vi "Saccade suppression - continuous flash LED.vi"() -> ()   [LabVIEW 2013]
uses:
  <vilib>/Platform/TimedLoop/XDataNode/timing_clust.ctl
  <vilib>/Platform/TimedLoop/XDataNode/nitl_modes.ctl
  <vilib>/Platform/TimedLoop/XDataNode/wakeup.ctl
  <vilib>/gmath/statdist.llb/Uniform (Discrete) Random.vi
  Eye tracking dependencies/Global 1.vi
  <vilib>/platform/TimedLoop/XDataNode/XDataNode.xnode
  <vilib>/Platform/TimedLoop/XDataNode/XDNodeRunTimeDep.lvlib
  <vilib>/gmath/NI_Gmath.lvlib
panel:
  out "Eye tracker":bool=TRUE
  out "Std name":string="70915_animal15-21_exp1"
  out "Blank":bool
  out "Total number of trials":i32=200
  out "Running!":bool
  in  "Location":string="D:\\Satoru\\Documents\\Attention_Beh_Data\\"
  out "File name exists!":bool
  out "Current trial #":u16
  out "LED":bool
  in  "Abort":bool caption="run-stop"
  in  "File name":string="animal15-29_exp1"
  in  "Save data":bool
  out "State Missed":bool
  out "VS missed":bool
  out "State busy":bool
  out "VS busy":bool
  in  "Tab Control":T1(tab)=enum."VS Parameters"
  in  "Notes":string
  in  "Start recording @":string
  in  "Inserted probe @":string
  in  "Brain region":string
  in  "Anesthesia @":string
  in  "Anesthesia":string
  in  "Probe configuration":string
  in  "Probe use number":string
  in  "Probe ID":string
  in  "Probe type":string
  in  "Electrode spacing":string
  in  "Electrode area":string
  in  "Penetration angle (to pia)":string
  in  "Penetration coordinates":string
  in  "Penetration distance":string
  in  "Penetration number":string
  in  "Genotype":string
  in  "Transfection":string
  in  "Mass":string
  in  "Sex":string
  in  "Age":string
  in  "Animal ID":string="14-4"
  in  "inter flash interval (ms)":dbl=300.0
  in  "Max jitter (ms)":dbl=250.0
  in  "VS type":string="continuous_flash"
  in  "Background luminance":sgl
  in  "Pulse amp 0":sgl
  in  "Pulse amp 1":sgl
  in  "Pulse delay (ms)":sgl
  in  "Pulse width (ms)":sgl
  in  "Pulse period":sgl
  in  "Pulse #":sgl
  in  "LED mode":u16(ring) items=["No LED", "Random"]
  in  "Chance (%)":dbl
  in  "# of trials":i32=200
  in  "run-stop":bool
  in  "movement":sgl=3.0
  in  "Flash luminance":sgl=100.0
  in  "flash duration (ms)":dbl=48.0
  in  "VS subtype":string="fullfield"
  in  "Include blanks":bool=TRUE
  in  "# of blank trials":i32=200
  in  "Give reward":bool
  in  "Manually give shock":bool
  in  "Water duration (ms)":u32=30
  in  "Shock duration (ms)":u32=10
  in  "Water refractory period (ms)":u32=500
  in  "Shock refractory period (ms)":u32=1000
  in  "Trial timeout (ms)":u32=3000
  in  "Track eye":bool=TRUE
  in  "Allow shock":bool
  in  "Allow timeout":bool
  in  "Manually give water":bool
  in  "Reward period (ms)":u32
  in  "Reward start delay (ms)":u32
  in  "Lick threshold (V)":fxp<+,32,16>=1.600006103515625
  in  "VS threshold (V)":fxp<+,32,16>=0.5
  out "Originating IP":string="192.168.137.2"
  out "Incoming data":string="TrlDone 1.000 "
  in  "Update cycle (ms)":dbl=50.0
  in  "Local IP_This computer":string="192.168.137.10"
  in  "Remote IP_Broadcast":string="192.168.137.255"
  in  "Remote IP_State machine":string="192.168.137.2"
  in  "Remote IP_Visual stimulation":string="192.168.137.3"
  in  "Local port":u16=9090
  in  "Remote port":u16=9091
  out "Error 2":string
  # "Saccade suppression project"
  # "Current trial"
  # "of"
  # "System Status"
  # "VS"
  # "State machine"
  # "Busy"
  # "Missed trial"
  # "Max 20 characters"
  # "(w/o LED)"
  # "Movement threshold (degrees)"
  # "MAX 199.9988"
  # "(% of blank trials that have LED)"
  # "Errors for debugging"
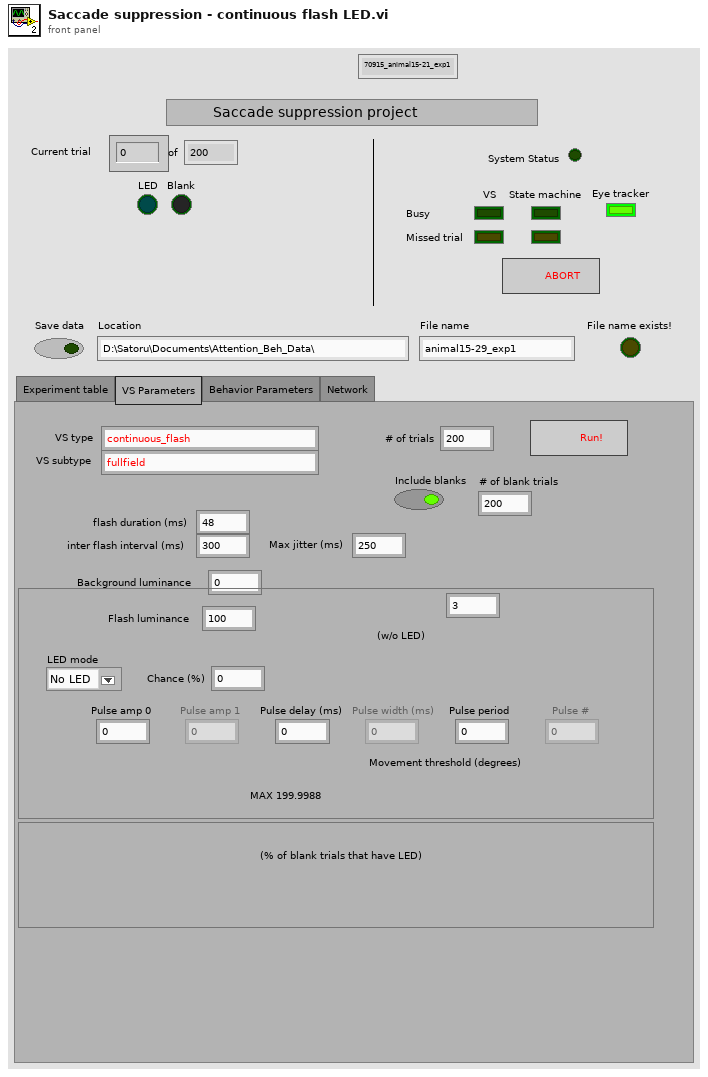
[diagram p1: front panel]
types:
  T1 = enum32{"Experiment table", "VS Parameters", "Behavior Parameters", "Network"}
  T2 = typedef "XDNodeRunTimeDep.lvlib/timing_clust.ctl" = cluster{"Expected End [f-1]":u64, "Actual End [f-1]":u64, "Finished Late? [f-1]":bool, "Expected End [i-1]":u64, "Actual End [i-1]":u64, "Finished Late? [i-1]":bool, "Expected Start [i]":u64, "Actual Start [i]":u64, "Expected Start [f]":u64, "Actual Start [f]":u64, "Source Name":string, "Structure Name":string, "Period":i64, "Deadline":i64, "Offset":i64, "Start":i64, "Priority":i32, "Timeout":i32, "Mode":T3, "Wakeup Reason":T4, "Error":errorcluster, "Source Type":string, "Secondary Source Type":string, "Global End Time":u64, "Global Start Time":u64, "Frame Duration":u64, "Iteration Duration":u64, "Assigned CPU":i32, "I/O Scan Engine Mode":u32}
  T3 = typedef "XDNodeRunTimeDep.lvlib/nitl_modes.ctl" = enum32{"No Change", "Process missed periods, maintain original phase", "Discard missed periods, maintain original phase", "Process missed periods, ignore original phase", "Discard missed periods, ignore original phase"}
  T4 = typedef "XDNodeRunTimeDep.lvlib/wakeup.ctl" = enum32{"Normal", "Aborted", "Asynchronous wakeup", "Timing source error", "Timed loop error", "Timeout"}
  T5 = enum16{"big-endian, network order", "native, host order", "little-endian"}
  T6 = enum16{"open", "replace", "create", "open or create", "replace or create", "replace or create with confirmation"}
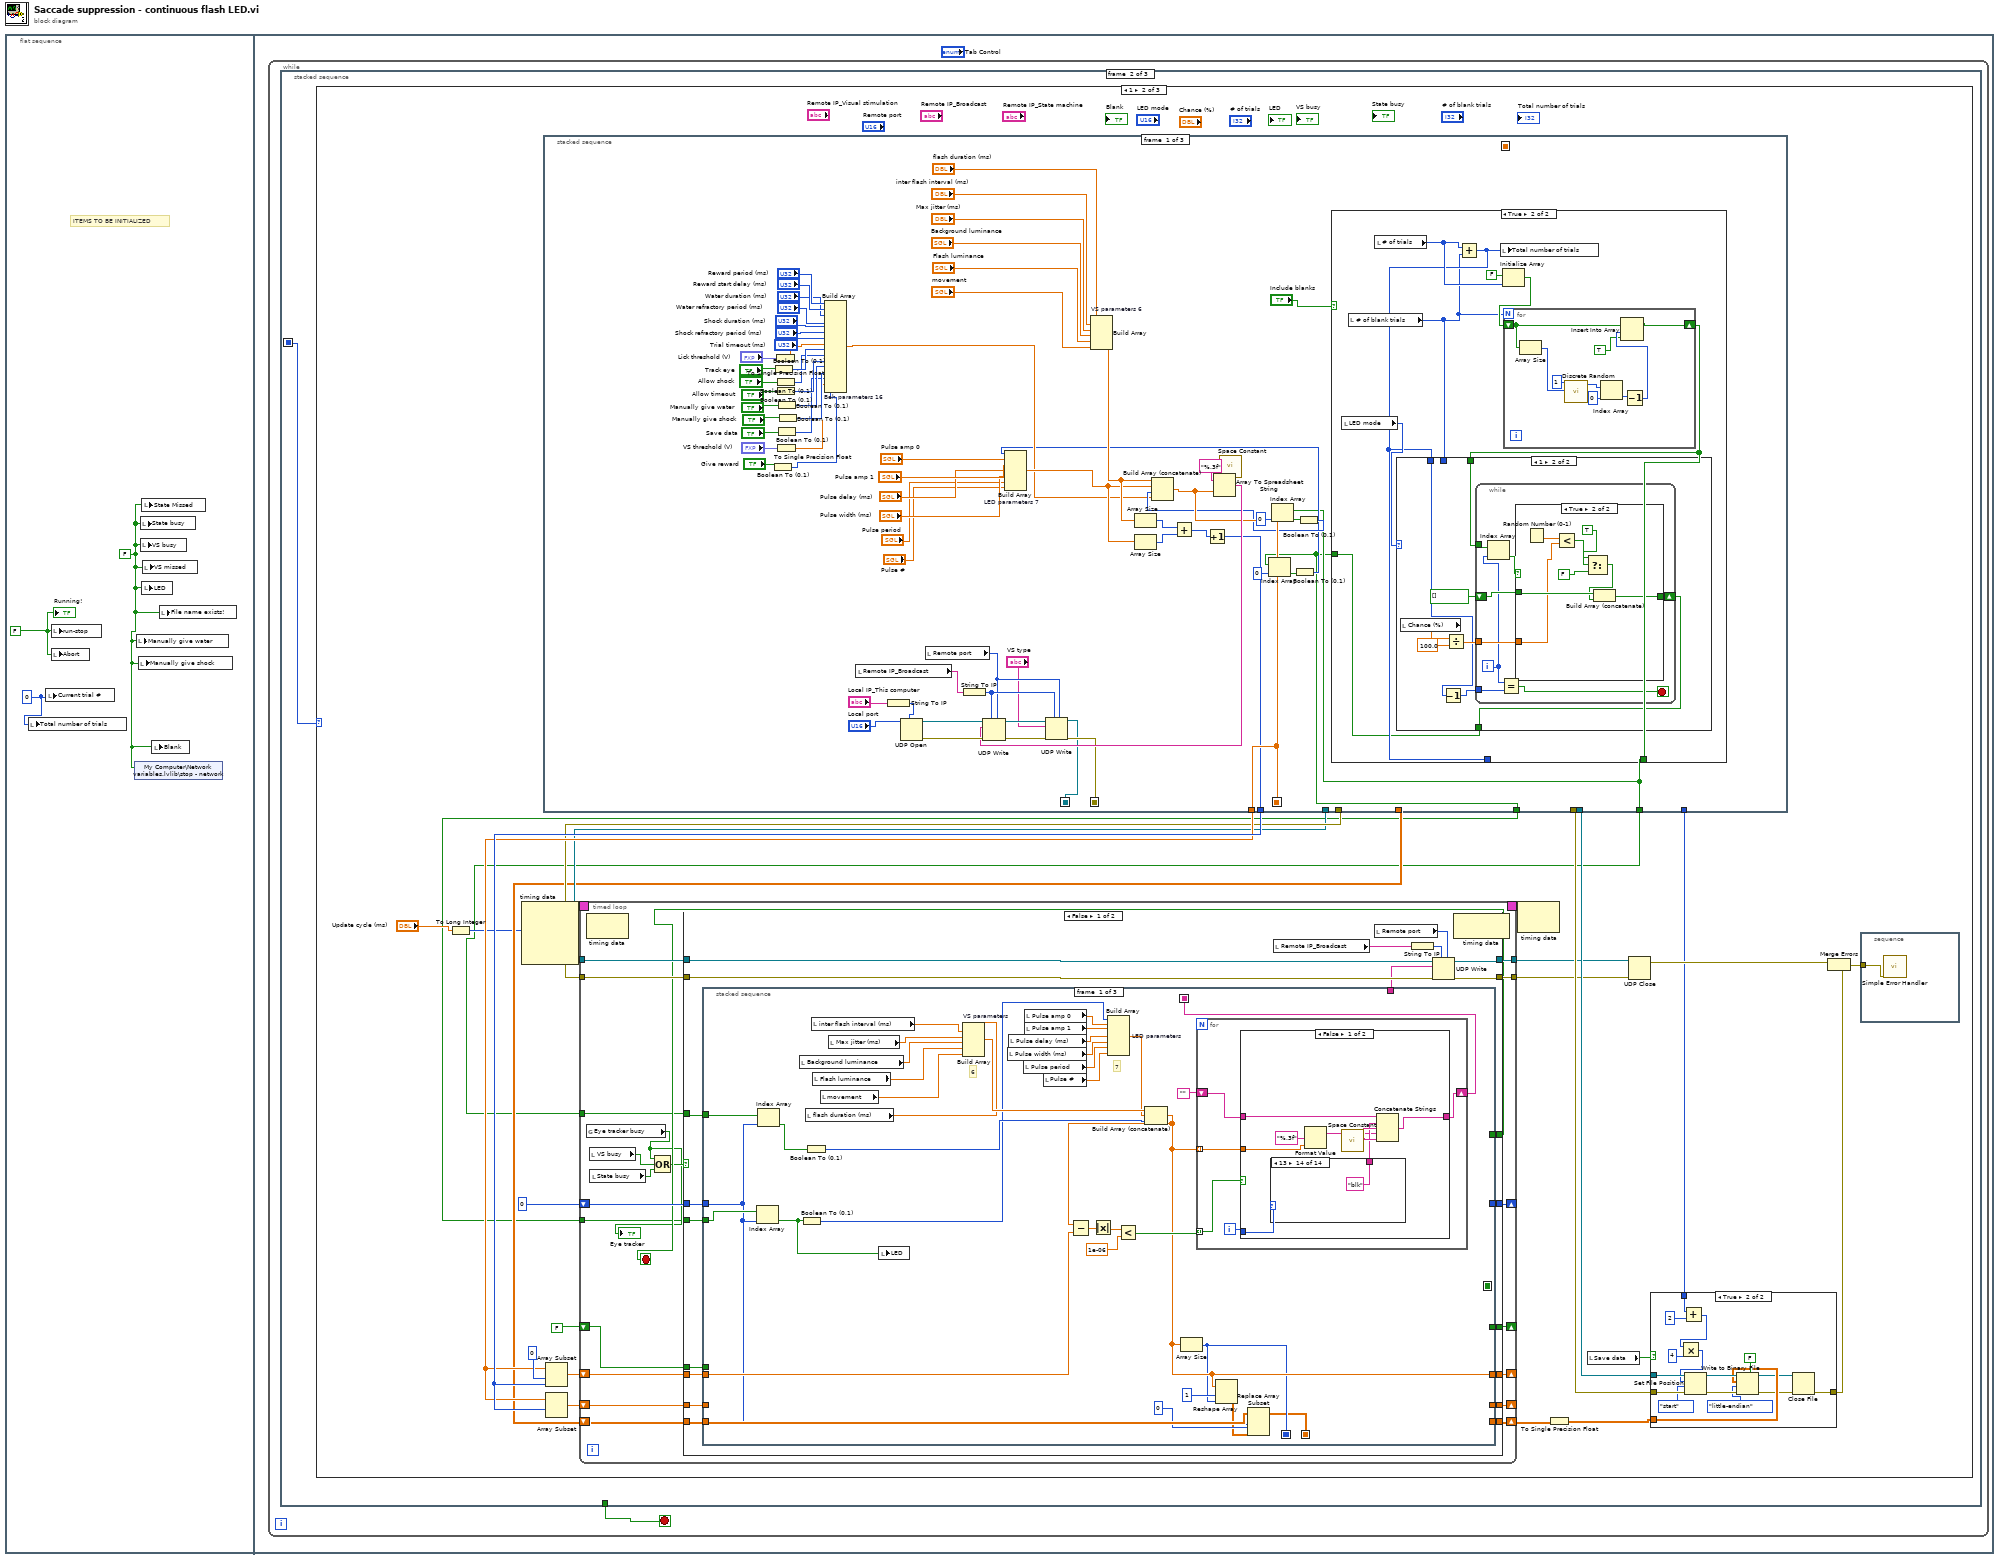
[diagram p0: block diagram]
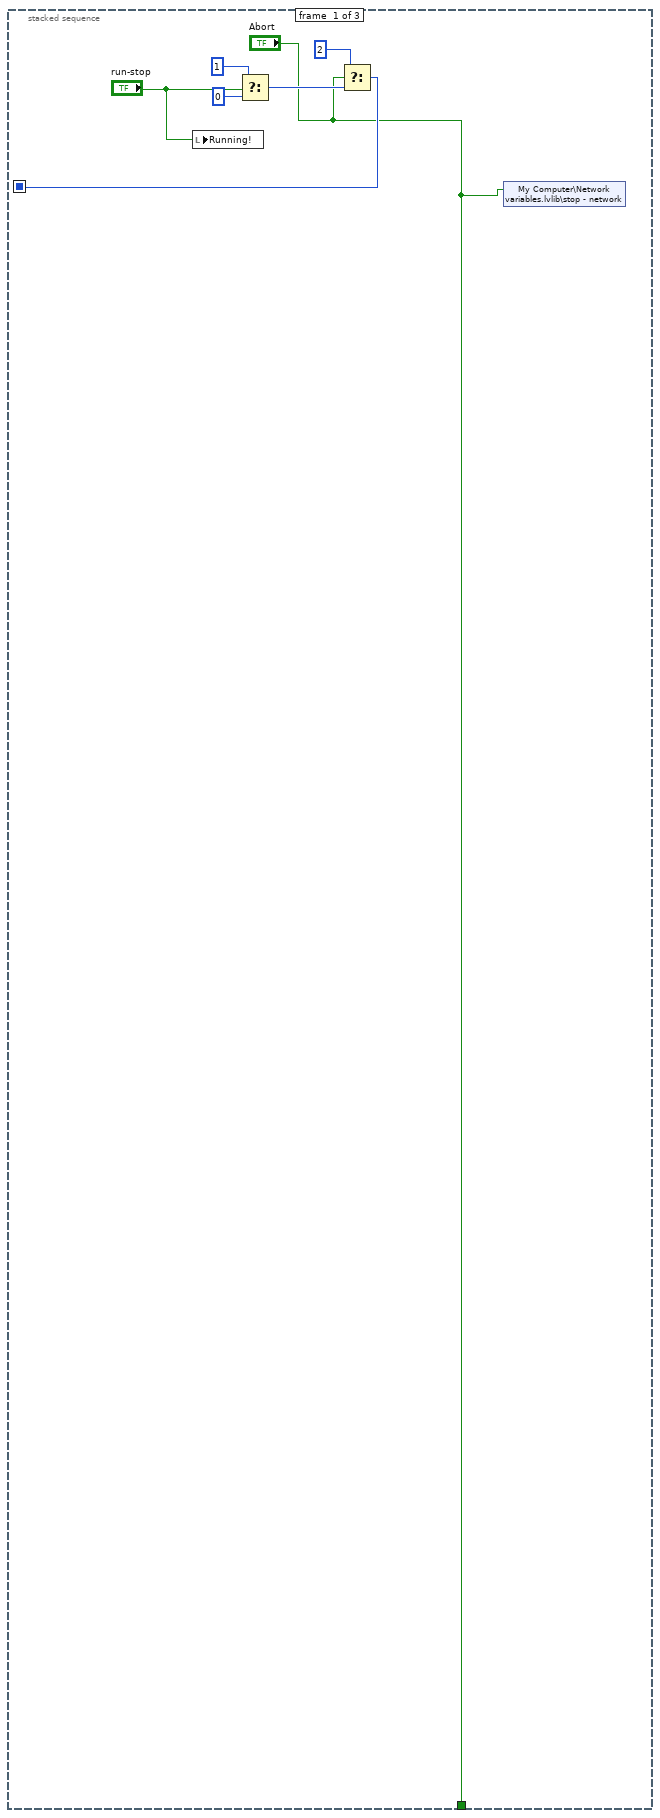
[diagram p2: hidden frame]
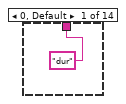
[diagram p4: hidden frame]
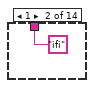
[diagram p5: hidden frame]
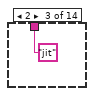
[diagram p6: hidden frame]
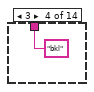
[diagram p7: hidden frame]
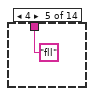
[diagram p8: hidden frame]
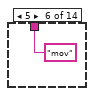
[diagram p9: hidden frame]
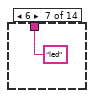
[diagram p10: hidden frame]
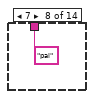
[diagram p11: hidden frame]
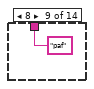
[diagram p12: hidden frame]
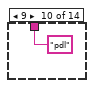
[diagram p13: hidden frame]
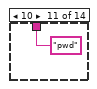
[diagram p14: hidden frame]
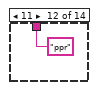
[diagram p15: hidden frame]
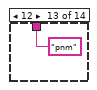
[diagram p16: hidden frame]
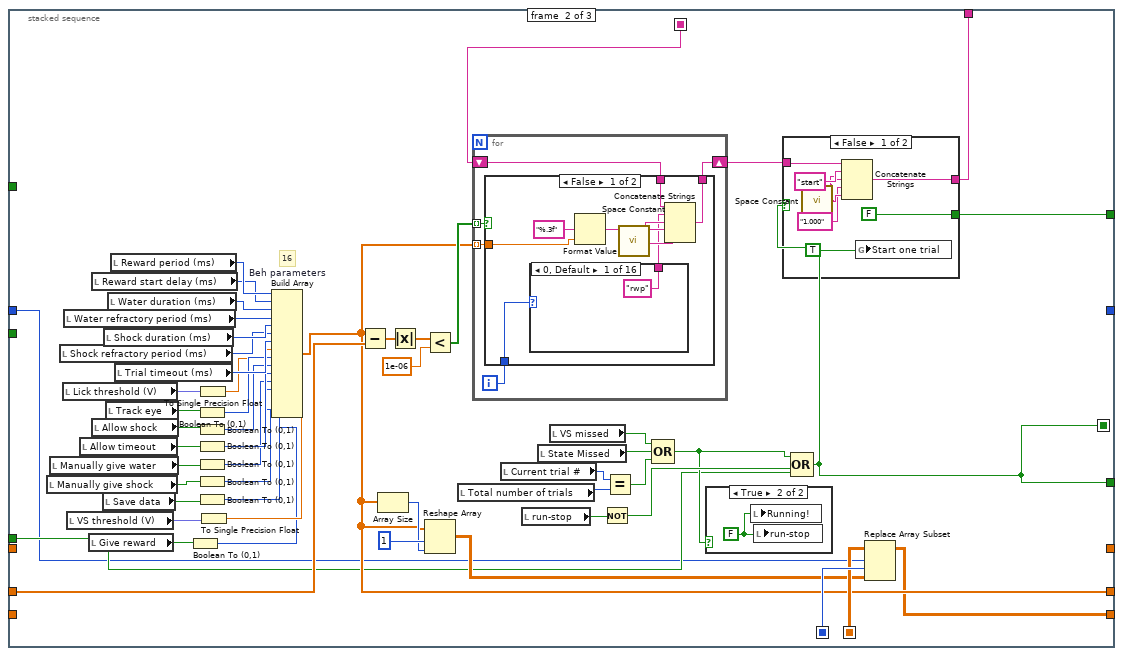
[diagram p18: hidden frame]
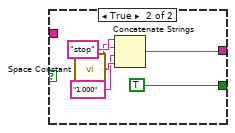
[diagram p20: hidden frame]
diagram:
  n1 = flat-sequence {
    frame #0 {
      w2 = u16 0
      w1 = FALSE ("L dist ind")
      w3 = FALSE
      # "ITEMS TO BE INITIALIZED"
      n2 = local write "Total number of trials"(w2) -> ()
      n3 = local write "Current trial #"(w2) -> ()
      n4 = local write "run-stop"(w3) -> ()
      n5 = local write "Abort"(w3) -> ()
      n6 = shared-variable "My Computer\\Network variables.lvlib\\stop - network"(w1) -> ()  [unwired: 1 in, 1 out]
      n7 = local write "Manually give water"(w1) -> ()
      n8 = local write "Manually give shock"(w1) -> ()
      n9 = local write "State busy"(w1) -> ()
      n10 = local write "VS busy"(w1) -> ()
      n11 = local write "State Missed"(w1) -> ()
      n12 = local write "LED"(w1) -> ()
      n13 = local write "VS missed"(w1) -> ()
      n14 = local write "Blank"(w1) -> ()
      n15 = local write "File name exists!"(w1) -> ()
      "Running!" <- w3
    }
    frame #1 {
      n16 = while {
        stop <- w4 stop-if-true
        n17 = stacked-sequence {
          seq-local: [w7 _ _] -> [_ w12 _]
          tunnel: ["Abort" _ _] -> w4
          frame #0 {
            n18 = local write "Running!"("run-stop") -> ()
            n19 = Select(t=u8 1, s="run-stop", f=u8 0) -> (s? t:f=w8:u8)
            n20 = Select(t=u8 2, s="Abort", f=w8) -> (s? t:f=w7:u8)
            n21 = shared-variable "My Computer\\Network variables.lvlib\\stop - network"("Abort") -> ()  [unwired: 1 in, 1 out]
          }
          frame #1 {
            n22 = case shown="1" w12 {
              frame 0, Default {
              }
              frame 1 {
                n23 = To Long Integer(number="Update cycle (ms)") -> (32bit integer=w22:i32)
                n24 = node-c288(w22) -> (w39:T2)  [unwired: 3 in]
                n25 = stacked-sequence {
                  seq-local: [w439 _ _] -> [_ _ w611]
                  seq-local: [_ w553 _] -> [_ _ w602]
                  seq-local: [w450 _ _] -> [_ _ w600]
                  seq-local: [w449 _ _] -> [_ _ w586]
                  tunnel: [w439 _ _] -> w34
                  tunnel: [w435 _ _] -> w35
                  tunnel: [_ _ w584] -> w31
                  tunnel: [_ _ w583] -> w30
                  tunnel: [_ _ w605] -> w29
                  tunnel: [_ _ w604] -> w25
                  tunnel: [_ _ w603] -> w24
                  tunnel: [_ _ w581] -> w15
                  tunnel: [w431 _ _] -> w14
                  tunnel: [w430 _ _] -> w13
                  frame #0 {
                    n26 = Boolean To (0,1)(Boolean="Give reward") -> (0, 1=w451:i16)
                    n27 = Boolean To (0,1)(Boolean="Track eye") -> (0, 1=w491:i16)
                    n28 = To Single Precision Float(number="Lick threshold (V)") -> (single precision float=w456:sgl)
                    n29 = Boolean To (0,1)(Boolean="Allow shock") -> (0, 1=w489:i16)
                    n30 = Boolean To (0,1)(Boolean="Allow timeout") -> (0, 1=w487:i16)
                    n31 = Boolean To (0,1)(Boolean="Manually give water") -> (0, 1=w485:i16)
                    n32 = Boolean To (0,1)(Boolean="Save data") -> (0, 1=w482:i16)
                    n33 = To Single Precision Float(number="VS threshold (V)") -> (single precision float=w453:sgl)
                    n34 = Boolean To (0,1)(Boolean="Manually give shock") -> (0, 1=w484:i16)
                    n35 = Build Array "Beh parameters 16"("Reward period (ms)", "Reward start delay (ms)", "Water duration (ms)", "Water refractory period (ms)", "Shock duration (ms)", "Shock refractory period (ms)", "Trial timeout (ms)", w456, w491, w489, w487, w485, w484, w482, w453, w451) -> (w437:sgl[])
                    n36 = local read "Remote IP_Broadcast"() -> (w469:string)
                    n37 = String To IP(1:"Local IP_This computer") -> (0:w473:u32)
                    n38 = UDP Open(7:w473, 11:"Local port") -> (port=w470:refnum<k16>, 0:w474:errorcluster)  [unwired: 3 in, 1 out]
                    n39 = local read "Remote port"() -> (w464:u16)
                    n40 = String To IP(1:w469) -> (0:w465:u32)
                    n41 = Build Array "VS parameters 6"("flash duration (ms)", "inter flash interval (ms)", "Max jitter (ms)", "Background luminance", "Flash luminance", "movement") -> (w460:dbl[])
                    n42 = Array Size(array=w460) -> (size(s)=w458:i32)
                    n43 = call <vilib>:"Space Constant.vi"() -> ("String"=w467:string)
                    n44 = case shown="True" "Include blanks" {
                      tunnel: [w503 w506] -> w431
                      tunnel: [w501 w508] -> _
                      tunnel: [w500 w507] -> w430
                      frame False {
                        n45 = local read "# of trials"() -> (w501:i32)
                        n46 = Initialize Array(FALSE, w501) -> (w500:bool[])
                        n47 = Initialize Array(FALSE, w501) -> (w503:bool[])
                        n48 = local write "Total number of trials"(w501) -> ()
                      }
                      frame True {
                        n49 = local read "LED mode"() -> (w509:u16)
                        n50 = local read "# of blank trials"() -> (w505:i32)
                        n51 = local read "# of trials"() -> (w510:i32)
                        n52 = Add(x=w510, y=w505) -> (x+y=w508:i32)
                        n53 = local write "Total number of trials"(w508) -> ()
                        n54 = Initialize Array(FALSE, w510) -> (w511:bool[])
                        n55 = for {
                          N: w505 -> [_]
                          shift-right: [w545] -> w506
                          shift-left: w511 -> [w546]
                          n56 = Array Size(array=w546) -> (size(s)=w550:i32)
                          n57 = call-poly <vilib>:"Discrete Random.vi"("n"=w550, "samples"=1) -> ("uniform (discrete) random data"=w549:i32[])  [unwired: 8 in, 1 out]
                          n58 = Index Array(array=w549, index=0) -> (element=w547:i32)
                          n59 = Decrement(x=w547) -> (x-1=w544:i32)
                          n60 = Insert Into Array(array=w546, index=w544, new element=TRUE) -> (w545:bool[])
                        }
                        n61 = case shown="1" w509 {
                          tunnel: w508 -> [w515 w517]
                          tunnel: [w514 w518] -> w507
                          tunnel: w506 -> [_ w523]
                          tunnel: w505 -> [_ _]
                          frame 0, Default {
                            n62 = Initialize Array(FALSE, w515) -> (w514:bool[])
                          }
                          frame 1 {
                            n63 = local read "Chance (%)"() -> (w521:dbl)
                            n64 = Decrement(x=w517) -> (x-1=w516:i32)
                            n65 = Divide(x=w521, y=100.0) -> (x/y=w519:dbl)
                            n66 = while {
                              tunnel: w523 -> [w531]
                              shift-right: [w529] -> w518
                              shift-left: bool[] [] -> [w528]
                              tunnel: w519 -> [w527]
                              tunnel: w516 -> [w525]
                              i -> [w526]
                              stop <- w524 stop-if-true
                              n67 = Index Array(array=w531, index=w526) -> (element=w530:bool)
                              n68 = Equal?(x=w526, y=w525) -> (x = y?=w524:bool)
                              n69 = case shown="True" w530 {
                                tunnel: [w533 w542] -> w529
                                tunnel: w528 -> [w532 w541]
                                tunnel: w527 -> [_ w536]
                                frame False {
                                n70 = Build Array (concatenate)(w532, FALSE) -> (w533:bool[])
                                }
                                frame True {
                                n71 = Random Number (0-1)() -> (number: 0 to 1=w535:dbl)
                                n72 = Less?(x=w535, y=w536) -> (x < y?=w537:bool)
                                n73 = Select(t=TRUE, s=w537, f=FALSE) -> (s? t:f=w540:bool)
                                n74 = Build Array (concatenate)(w541, w540) -> (w542:bool[])
                                }
                              }
                            }
                          }
                        }
                      }
                    }
                    n75 = Index Array(array=w430, index=0) -> (element=w433:bool)
                    n76 = Index Array(array=w431, index=0) -> (element=w440:bool)
                    n77 = Boolean To (0,1)(Boolean=w433) -> (0, 1=w432:i16)
                    n78 = Build Array "LED parameters 7"(w432, "Pulse amp 0", "Pulse amp 1", "Pulse delay (ms)", "Pulse width (ms)", "Pulse period", "Pulse #") -> (w459:sgl[])
                    n79 = Array Size(array=w459) -> (size(s)=w457:i32)
                    n80 = Add(x=w458, y=w457) -> (x+y=w436:i32)
                    n81 = Increment(x=w436) -> (x+1=w435:i32)
                    n82 = Boolean To (0,1)(Boolean=w440) -> (0, 1=w438:i16)
                    n83 = Build Array (concatenate)(w460, w459, w438, w437) -> (w439:dbl[])
                    n84 = Array To Spreadsheet String(delimiter (Tab)=w467, array=w439, 3:"%.3f" ("format string")) -> (spreadsheet string=w466:string)
                    n85 = UDP Write(address=w465, port or service name=w464, connection ID=w470, data in=w466, 8:w474) -> (error out=w463:errorcluster, 3:w462:refnum<k16>)  [unwired: 1 in]
                    n86 = UDP Write(address=w465, port or service name=w464, connection ID=w462, data in="VS type", 8:w463) -> (error out=w450:errorcluster, 3:w449:refnum<k16>)  [unwired: 1 in]
                  }
                  frame #1 {
                    w560 = "&" ("string")
                    # "state definition"
                    n87 = local read "inter flash interval (ms)"() -> (w575:dbl)
                    n88 = local read "Total number of trials"() -> (w552:i32)
                    n89 = local read "Max jitter (ms)"() -> (w574:dbl)
                    n90 = local read "VS subtype"() -> (w579:string)
                    n91 = local read "Chance (%)"() -> (w573:dbl)
                    n92 = local read "LED mode"() -> (w576:u16)
                    n93 = local read "VS type"() -> (w580:string)
                    n94 = String To Byte Array(string=w580) -> (unsigned byte array=w578:u8[])
                    n95 = String To Byte Array(string=w579) -> (unsigned byte array=w577:u8[])
                    n96 = Concatenate Strings("idle", w560, "vs before", w560, "vs", w560, "vs after", w560, "cycle end", w560, "reward", w560, "reward refractory", w560, "punish", w560, "punish refractory", w560, "exit", w560, "timeout", w560) -> (w561:string)
                    n97 = Build Array (concatenate)(w578, w577, w576, w552, w575, w574, w573) -> (w557:dbl[])
                    n98 = String To Byte Array(string=w561) -> (unsigned byte array=w555:u8[])
                    n99 = Initialize Array(sgl 0.0 ("element"), 37 ("dimension size")) -> (w556:sgl[])
                    n100 = Build Array (concatenate)(w557, w556, w555) -> (w554:dbl[])
                    n101 = To Single Precision Float(number=w554) -> (single precision float=w553:sgl[])
                  }
                  frame #2 {
                    # "# of parameters, column"
                    n102 = local read "Save data"() -> (w608:bool)
                    n103 = local read "Remote IP_Broadcast"() -> (w594:string)
                    n104 = local read "Remote port"() -> (w592:u16)
                    n105 = String To IP(1:w594) -> (0:w593:u32)
                    n106 = local read "Total number of trials"() -> (w601:i32)
                    n107 = Array Size(array=w611) -> (size(s)=w609:i32)
                    n108 = Build Array(w601, w609) -> (w607:i32[])
                    n109 = Initialize Array(sgl 0.0, w601, w609) -> (w605:sgl[][])
                    n110 = To Single Precision Float(number=w607) -> (single precision float=w606:sgl[])
                    n111 = case shown="True" w608 {
                      tunnel: w606 -> [_ w684]
                      tunnel: w605 -> [_ w683]
                      tunnel: [_ w682] -> w604
                      tunnel: [_ w681] -> w603
                      tunnel: w602 -> [_ w680]
                      tunnel: ["" w616] -> w588
                      tunnel: [_ w615] -> w581
                      frame False {
                      }
                      frame True {
                        w651 = 20 ("dimension size")
                        w621 = 500 ("dimension size")
                        w623 = T5."little-endian" ("byte order (0:big-endian, network order)")
                        w693 = enum16{"start", "end", "current"}."start" ("from (0:start)")
                        # "param array"
                        # "row and col\nfor param array"
                        # "first 500 singles for common params"
                        # "reserve 500 singles"
                        # "write behhavior params"
                        # "datapath"
                        n112 = while {
                          tunnel: [w724] -> w686
                          tunnel: [w723] -> w685
                          tunnel: [w716] -> w616
                          stop <- w721 continue-if-true
                          (unwired) "0" ("replace string (\"\")")
                          w745 = "/"
                          n113 = Get Date/Time String() -> (date string=w747:string)  [unwired: 3 in, 1 out]
                          n114 = Match Pattern(string=w747, regular expression=w745) -> (before substring=w744:string, after substring=w746:string)  [unwired: 1 in, 2 out]
                          n115 = Decimal String To Number(string=w744) -> (number=w739:i32)  [unwired: 2 in, 1 out]
                          n116 = Match Pattern(string=w746, regular expression=w745) -> (before substring=w743:string, after substring=w733:string)  [unwired: 1 in, 2 out]
                          n117 = Number To Decimal String(number=w739, width (-)=i16 2) -> (decimal integer string=w741:string)
                          n118 = call <vilib>:"Space Constant.vi"() -> ("String"=w740:string)
                          n119 = Decimal String To Number(string=w743) -> (number=w736:i32)  [unwired: 2 in, 1 out]
                          n120 = Search and Replace String(input string=w741, search string=w740) -> (result string=w731:string)  [unwired: 6 in, 3 out]
                          n121 = Number To Decimal String(number=w736, width (-)=i16 2) -> (decimal integer string=w738:string)
                          n122 = String Subset(string=w733, offset (0)=2) -> (substring=w729:string)  [unwired: 1 in]
                          n123 = call <vilib>:"Space Constant.vi"() -> ("String"=w737:string)
                          n124 = Search and Replace String(input string=w738, search string=w737, replace string="0" ("replace string (\"\")")) -> (result string=w730:string)  [unwired: 5 in, 3 out]
                          n125 = Concatenate Strings(w731, w730, w729) -> (w719:string)
                          n126 = Concatenate Strings(w719, "_" ("string"), "File name") -> (w716:string)
                          "Std name" <- w716
                          n127 = Concatenate Strings("Location", w719, "_" ("string"), "File name", ".beh" ("string")) -> (w726:string)
                          n128 = Wait (ms)(milliseconds to wait=u32 100) -> ()  [unwired: 1 out]
                          n129 = String To Path(string=w726) -> (path=w725:path)
                          n130 = call <vilib>:"Check if File or Folder Exists.vi"("path"=w725) -> ("error out"=w723:errorcluster, "file or folder exists?"=w721:bool, "dup path"=w724:path)  [unwired: 8 in]
                          "File name exists!" <- w721
                        }
                        n131 = String To Byte Array(string="Animal ID") -> (unsigned byte array=w643:u8[])
                        n132 = String To Byte Array(string="Genotype") -> (unsigned byte array=w634:u8[])
                        n133 = String To Byte Array(string="Age") -> (unsigned byte array=w635:u8[])
                        n134 = String To Byte Array(string="Sex") -> (unsigned byte array=w636:u8[])
                        n135 = String To Byte Array(string="Mass") -> (unsigned byte array=w637:u8[])
                        n136 = String To Byte Array(string="Transfection") -> (unsigned byte array=w638:u8[])
                        n137 = String To Byte Array(string="Penetration number") -> (unsigned byte array=w640:u8[])
                        n138 = String To Byte Array(string="Penetration distance") -> (unsigned byte array=w642:u8[])
                        n139 = String To Byte Array(string="Penetration coordinates") -> (unsigned byte array=w666:u8[])
                        n140 = String To Byte Array(string="Penetration angle (to pia)") -> (unsigned byte array=w667:u8[])
                        n141 = String To Byte Array(string="Electrode area") -> (unsigned byte array=w668:u8[])
                        n142 = String To Byte Array(string="Electrode spacing") -> (unsigned byte array=w669:u8[])
                        n143 = String To Byte Array(string="Probe type") -> (unsigned byte array=w670:u8[])
                        n144 = String To Byte Array(string="Probe ID") -> (unsigned byte array=w671:u8[])
                        n145 = String To Byte Array(string="Probe use number") -> (unsigned byte array=w672:u8[])
                        n146 = String To Byte Array(string="Probe configuration") -> (unsigned byte array=w673:u8[])
                        n147 = String To Byte Array(string="Anesthesia") -> (unsigned byte array=w674:u8[])
                        n148 = String To Byte Array(string="Anesthesia @") -> (unsigned byte array=w675:u8[])
                        n149 = String To Byte Array(string="Brain region") -> (unsigned byte array=w676:u8[])
                        n150 = String To Byte Array(string="Inserted probe @") -> (unsigned byte array=w677:u8[])
                        n151 = String To Byte Array(string="Start recording @") -> (unsigned byte array=w678:u8[])
                        n152 = String To Byte Array(string="Notes") -> (unsigned byte array=w679:u8[])
                        n153 = Build Array(w643, w634, w635, w636, w637, w638, w640, w642, w666, w667, w668, w669, w670, w671, w672, w673, w674, w675, w676, w677, w678, w679) -> (w646:u8[][])
                        n154 = for {
                          tunnel: w646 -> [w713] mode=indexing
                          tunnel: [w712] -> w644 mode=indexing
                          tunnel: w651 -> [w711]
                          n155 = Initialize Array(u8 0 ("element"), w711) -> (w715:u8[])
                          n156 = Replace Array Subset(array=w715, new element=w713) -> (w712:u8[])  [unwired: 1 in]
                        }
                        n157 = Array Size(array=w646) -> (size(s)=w648:i32[])
                        n158 = Index Array(array=w648, index=0) -> (element=w650:i32)
                        n159 = Open/Create/Replace File(file path (use dialog)=w686, error in=w685, operation (0:open)=T6."create", access (0:read/write)=enum16{"read/write", "read-only", "write-only"}."write-only") -> (refnum out=w707:refnum<file>, error out=w706:errorcluster)  [unwired: 2 in, 1 out]
                        n160 = Multiply(x=w651, y=w650) -> (x*y=w619:i32)
                        n161 = Set File Position(offset (in bytes) (0)=i64 0, refnum=w707, from (0:start)=w693, error in=w706) -> (refnum out=w627:refnum<file>, error out=w625:errorcluster)
                        n162 = To Single Precision Float(number=w644) -> (single precision float=w645:sgl[][])
                        n163 = Initialize Array(sgl 0.0 ("element"), w621) -> (w703:sgl[])
                        n164 = Reshape Array(w645, 1 ("dimension size"), w619) -> (w622:sgl[][])
                        n165 = Write to Binary File(file (use dialog)=w627, data=w622, error in=w625, 5:FALSE ("prepend array or string size? (T)"), 9:w623) -> (refnum out=w626:refnum<file>, error out=w624:errorcluster)  [unwired: 1 in, 1 out]
                        n166 = Write to Binary File(file (use dialog)=w626, data=w703, error in=w624, 5:FALSE ("prepend array or string size? (T)"), 9:w623) -> (refnum out=w701:refnum<file>, error out=w700:errorcluster)  [unwired: 1 in, 1 out]
                        n167 = Multiply(x=w619, y=4) -> (x*y=w620:i32)
                        n168 = Set File Position(offset (in bytes) (0)=w620, refnum=w701, from (0:start)=w693, error in=w700) -> (refnum out=w699:refnum<file>, error out=w698:errorcluster)
                        n169 = Add(x=w619, y=w621) -> (x+y=w615:i32)
                        n170 = Write to Binary File(file (use dialog)=w699, data=w680, error in=w698, 5:FALSE ("prepend array or string size? (T)"), 9:w623) -> (refnum out=w697:refnum<file>, error out=w696:errorcluster)  [unwired: 1 in, 1 out]
                        n171 = Multiply(x=w615, y=4) -> (x*y=w695:i32)
                        n172 = Set File Position(offset (in bytes) (0)=w695, refnum=w697, from (0:start)=w693, error in=w696) -> (refnum out=w691:refnum<file>, error out=w690:errorcluster)
                        n173 = Write to Binary File(file (use dialog)=w691, data=w684, error in=w690, 5:FALSE ("prepend array or string size? (T)"), 9:w623) -> (refnum out=w689:refnum<file>, error out=w688:errorcluster)  [unwired: 1 in, 1 out]
                        n174 = Write to Binary File(file (use dialog)=w689, data=w683, error in=w688, 5:FALSE ("prepend array or string size? (T)"), 9:w623) -> (refnum out=w681:refnum<file>, error out=w682:errorcluster)  [unwired: 1 in, 1 out]
                      }
                    }
                    n175 = String Length(string=w588) -> (length=w591:i32)
                    n176 = Not Equal To 0?(x=w591) -> (x != 0?=w590:bool)
                    n177 = Select(t=w588, s=w590, f="Test") -> (s? t:f=w587:string)
                    n178 = UDP Write(address=w593, port or service name=w592, connection ID=w586, data in=w587, 8:w600) -> (error out=w599:errorcluster, 3:w585:refnum<k16>)  [unwired: 1 in]
                    n179 = UDP Write(address=w593, port or service name=w592, connection ID=w585, data in="VS subtype", 8:w599) -> (error out=w595:errorcluster, 3:w583:refnum<k16>)  [unwired: 1 in]
                    n180 = Unbundle By Name(w595) -> ("code"=w598:i32)
                    n181 = Equal?(x=w598, y=56) -> (x = y?=w596:bool)
                    n182 = case shown="True" w596 {
                      tunnel: w595 -> [w612 _]
                      tunnel: [w612 errorcluster {"status"=FALSE, "code"=0, "source"=""} ("error out")] -> w584
                      frame False {
                      }
                      frame True {
                      }
                    }
                  }
                }
                n183 = Array Subset(array=w34, index=0, length=w35) -> (w37:dbl[])
                n184 = Array Subset(array=w34, index=w35) -> (w33:dbl[])  [unwired: 1 in]
                n185 = timed-loop {
                  shift-right: [w59] -> _
                  shift-left: u16 0 -> [w58]
                  tunnel: w31 -> [w57]
                  tunnel: w30 -> [w56]
                  tunnel: [w55] -> w16
                  tunnel: [w54] -> w17
                  shift-right: [w53] -> _
                  shift-left: w37 -> [w61]
                  shift-right: [w52] -> _
                  shift-left: w33 -> [w60]
                  shift-right: [w50] -> w28
                  shift-left: w29 -> [w51]
                  shift-right: [w49] -> _
                  shift-left: FALSE -> [w48]
                  timing: w39 -> [_]
                  timing-out: [_] -> w38
                  tunnel: w14 -> [w42]
                  tunnel: w13 -> [w41]
                  stop <- w47 stop-if-true
                  n186 = node-c288() -> ()  [unwired: 1 in, 1 out]
                  n187 = global read "Global 1.vi" "Eye tracker busy"() -> (w43:bool)
                  "Eye tracker" <- w43
                  n188 = local read "VS busy"() -> (w45:bool)
                  n189 = local read "State busy"() -> (w44:bool)
                  n190 = Compound Arithmetic op=OR(w43, w45, w44) -> (w46:bool)
                  n191 = case shown="False" w46 {
                    tunnel: w61 -> [w84 w262]
                    tunnel: w60 -> [w83 w260]
                    tunnel: [w82 w251] -> w59
                    tunnel: w58 -> [w81 w252]
                    tunnel: w57 -> [w77 w258]
                    tunnel: w56 -> [w76 w256]
                    tunnel: [w75 w257] -> w55
                    tunnel: [w74 w255] -> w54
                    tunnel: [w73 w262] -> w53
                    tunnel: [w72 w253] -> w52
                    tunnel: w51 -> [w71 w261]
                    tunnel: [w70 w261] -> w50
                    tunnel: [w69 w254] -> w49
                    tunnel: w48 -> [w68 w259]
                    tunnel: [w66 FALSE] -> w47
                    tunnel: w42 -> [w65 _]
                    tunnel: w41 -> [w64 _]
                    frame False {
                      n192 = stacked-sequence {
                        seq-local: [w106 _ _] -> [_ w173 _]
                        seq-local: [w99 _ _] -> [_ w167 _]
                        seq-local: [w98 _ _] -> [_ w166 _]
                        seq-local: [_ w156 _] -> [_ _ w243]
                        tunnel: w81 -> [w87 w154 w245]
                        tunnel: w84 -> [w111 _ _]
                        tunnel: w83 -> [_ w180 _]
                        tunnel: [_ _ w244] -> w82
                        tunnel: [w103 _ _] -> w73
                        tunnel: [_ w163 _] -> w72
                        tunnel: w71 -> [w102 _ _]
                        tunnel: [_ w161 _] -> w70
                        tunnel: [_ w156 _] -> w69
                        tunnel: w68 -> [_ w157 _]
                        tunnel: [_ w155 _] -> w67
                        tunnel: [_ w148 _] -> w66
                        tunnel: w65 -> [w91 _ _]
                        tunnel: w64 -> [w88 _ _]
                        frame #0 {
                          # "6"
                          # "7"
                          n193 = Index Array(array=w88, index=w87) -> (element=w85:bool)
                          n194 = Index Array(array=w91, index=w87) -> (element=w90:bool)
                          n195 = local read "Background luminance"() -> (w95:sgl)
                          n196 = Boolean To (0,1)(Boolean=w85) -> (0, 1=w86:i16)
                          n197 = Boolean To (0,1)(Boolean=w90) -> (0, 1=w89:i16)
                          n198 = local read "flash duration (ms)"() -> (w92:dbl)
                          n199 = local read "inter flash interval (ms)"() -> (w97:dbl)
                          n200 = local read "Flash luminance"() -> (w94:sgl)
                          n201 = local read "movement"() -> (w93:sgl)
                          n202 = local read "Max jitter (ms)"() -> (w96:dbl)
                          n203 = local write "LED"(w85) -> ()
                          n204 = Build Array "VS parameters"(w92, w97, w96, w95, w94, w93) -> (w113:dbl[])
                          n205 = local read "Pulse width (ms)"() -> (w117:sgl)
                          n206 = local read "Pulse delay (ms)"() -> (w116:sgl)
                          n207 = local read "Pulse period"() -> (w118:sgl)
                          n208 = local read "Pulse amp 0"() -> (w114:sgl)
                          n209 = local read "Pulse amp 1"() -> (w115:sgl)
                          n210 = local read "Pulse #"() -> (w119:sgl)
                          n211 = Build Array "LED parameters"(w86, w114, w115, w116, w117, w118, w119) -> (w112:sgl[])
                          n212 = Build Array (concatenate)(w113, w112, w89) -> (w103:dbl[])
                          n213 = Subtract(x=w103, y=w111) -> (x-y=w110:dbl[])
                          n214 = Absolute Value(x=w110) -> (abs(x)=w108:dbl[])
                          n215 = Less?(x=w108, y=1e-06) -> (x < y?=w107:bool[])
                          n216 = Array Size(array=w103) -> (size(s)=w99:i32)
                          n217 = for {
                            tunnel: w107 -> [w124] mode=indexing
                            shift-right: [w122] -> w106
                            shift-left: "" -> [w123]
                            tunnel: w103 -> [w121] mode=indexing
                            i -> [w120]
                            n218 = case shown="False" w124 {
                              tunnel: w123 -> [w132 w147]
                              tunnel: [w131 w147] -> w122
                              tunnel: w120 -> [w129 _]
                              tunnel: w121 -> [w125 _]
                              frame False {
                                n219 = case shown="13" w129 {
                                tunnel: ["dur" "ifi" "jit" "bkl" "fll" "mov" "led" "pai" "paf" "pdl" "pwd" "ppr" "pnm" "blk"] -> w128
                                frame 0, Default {
                                }
                                frame 1 {
                                }
                                frame 2 {
                                }
                                frame 3 {
                                }
                                frame 4 {
                                }
                                frame 5 {
                                }
                                frame 6 {
                                }
                                frame 7 {
                                }
                                frame 8 {
                                }
                                frame 9 {
                                }
                                frame 10 {
                                }
                                frame 11 {
                                }
                                frame 12 {
                                }
                                frame 13 {
                                }
                                }
                                n220 = Format Value(format string="%.3f", value (0)=w125) -> (output string=w126:string)  [unwired: 1 in]
                                n221 = call <vilib>:"Space Constant.vi"() -> ("String"=w130:string)
                                n222 = Concatenate Strings(w132, w128, w130, w126, w130) -> (w131:string)
                              }
                              frame True {
                              }
                            }
                          }
                          n223 = Reshape Array(w103, 1 ("dimension size"), w99) -> (w100:dbl[][])
                          n224 = Replace Array Subset(array=w102, new element=w100, index (row)=w87, index (col)=0) -> (w98:sgl[][])
                        }
                        frame #1 {
                          # "16"
                          n225 = local read "Manually give shock"() -> (w184:bool)
                          n226 = local read "Manually give water"() -> (w186:bool)
                          n227 = local read "Shock refractory period (ms)"() -> (w194:u32)
                          n228 = local read "Lick threshold (V)"() -> (w174:fxp<+,32,16>)
                          n229 = local read "Water refractory period (ms)"() -> (w196:u32)
                          n230 = local read "VS threshold (V)"() -> (w152:fxp<+,32,16>)
                          n231 = local read "Allow timeout"() -> (w188:bool)
                          n232 = local read "Give reward"() -> (w150:bool)
                          n233 = local read "Reward start delay (ms)"() -> (w198:u32)
                          n234 = local read "Allow shock"() -> (w190:bool)
                          n235 = local read "Save data"() -> (w182:bool)
                          n236 = local read "Shock duration (ms)"() -> (w195:u32)
                          n237 = local read "Track eye"() -> (w191:bool)
                          n238 = local read "Water duration (ms)"() -> (w197:u32)
                          n239 = local read "Reward period (ms)"() -> (w199:u32)
                          n240 = local read "Trial timeout (ms)"() -> (w193:u32)
                          n241 = Boolean To (0,1)(Boolean=w150) -> (0, 1=w149:i16)
                          n242 = Boolean To (0,1)(Boolean=w191) -> (0, 1=w192:i16)
                          n243 = Boolean To (0,1)(Boolean=w190) -> (0, 1=w189:i16)
                          n244 = Boolean To (0,1)(Boolean=w188) -> (0, 1=w187:i16)
                          n245 = Boolean To (0,1)(Boolean=w186) -> (0, 1=w185:i16)
                          n246 = Boolean To (0,1)(Boolean=w184) -> (0, 1=w183:i16)
                          n247 = Boolean To (0,1)(Boolean=w182) -> (0, 1=w181:i16)
                          n248 = To Single Precision Float(number=w174) -> (single precision float=w175:sgl)
                          n249 = To Single Precision Float(number=w152) -> (single precision float=w151:sgl)
                          n250 = Build Array "Beh parameters"(w199, w198, w197, w196, w195, w194, w193, w175, w192, w189, w187, w185, w183, w181, w151, w149) -> (w163:sgl[])
                          n251 = Subtract(x=w163, y=w180) -> (x-y=w179:dbl[])
                          n252 = Array Size(array=w163) -> (size(s)=w164:i32)
                          n253 = Absolute Value(x=w179) -> (abs(x)=w177:dbl[])
                          n254 = Less?(x=w177, y=1e-06) -> (x < y?=w176:bool[])
                          n255 = Reshape Array(w163, 1 ("dimension size"), w164) -> (w162:sgl[][])
                          n256 = local read "Total number of trials"() -> (w153:i32)
                          n257 = for {
                            tunnel: w176 -> [w216] mode=indexing
                            tunnel: w163 -> [w215] mode=indexing
                            shift-right: [w213] -> w172
                            shift-left: w173 -> [w214]
                            i -> [w217]
                            n258 = case shown="False" w216 {
                              tunnel: w217 -> [w225 _]
                              tunnel: w215 -> [w223 _]
                              tunnel: w214 -> [w220 w242]
                              tunnel: [w218 w242] -> w213
                              frame False {
                                n259 = case shown="0, Default" w225 {
                                tunnel: ["rwp" "rwd" "wdr" "wre" "shd" "shr" "tto" "lkt" "etk" "ash" "ato" "gwt" "gsh" "sav" "vsh" "rew"] -> w219
                                frame 0, Default {
                                }
                                frame 1 {
                                }
                                frame 2 {
                                }
                                frame 3 {
                                }
                                frame 4 {
                                }
                                frame 5 {
                                }
                                frame 6 {
                                }
                                frame 7 {
                                }
                                frame 8 {
                                }
                                frame 9 {
                                }
                                frame 10 {
                                }
                                frame 11 {
                                }
                                frame 12 {
                                }
                                frame 13 {
                                }
                                frame 14 {
                                }
                                frame 15 {
                                }
                                }
                                n260 = Format Value(format string="%.3f", value (0)=w223) -> (output string=w221:string)  [unwired: 1 in]
                                n261 = call <vilib>:"Space Constant.vi"() -> ("String"=w222:string)
                                n262 = Concatenate Strings(w220, w219, w222, w221, w222) -> (w218:string)
                              }
                              frame True {
                              }
                            }
                          }
                          n263 = local read "Current trial #"() -> (w168:u16)
                          n264 = local read "run-stop"() -> (w160:bool)
                          n265 = local read "State Missed"() -> (w170:bool)
                          n266 = local read "VS missed"() -> (w169:bool)
                          n267 = Not(x=w160) -> (.not. x?=w159:bool)
                          n268 = Equal?(x=w168, y=w153) -> (x = y?=w171:bool)
                          n269 = Compound Arithmetic op=OR(w169, w170, w171) -> (w158:bool)
                          n270 = case shown="True" w158 {
                            frame False {
                            }
                            frame True {
                              w200 = FALSE
                              n271 = local write "Running!"(w200) -> ()
                              n272 = local write "run-stop"(w200) -> ()
                            }
                          }
                          n273 = Compound Arithmetic op=OR(w158, w159, w157) -> (w156:bool)
                          n274 = case shown="False" w156 {
                            tunnel: w172 -> [w207 _]
                            tunnel: [w203 w209] -> w155
                            tunnel: [FALSE TRUE] -> w148
                            frame False {
                              n275 = call <vilib>:"Space Constant.vi"() -> ("String"=w205:string)
                              n276 = Concatenate Strings(w207, "start", w205, "1.000", w205) -> (w203:string)
                              n277 = global write "Global 1.vi" "Start one trial"(TRUE) -> ()
                            }
                            frame True {
                              n278 = call <vilib>:"Space Constant.vi"() -> ("String"=w211:string)
                              n279 = Concatenate Strings("stop", w211, "1.000", w211) -> (w209:string)
                            }
                          }
                          n280 = Replace Array Subset(array=w166, new element=w162, index (row)=w154, index (col)=w167) -> (w161:sgl[][])
                        }
                        frame #2 {
                          n281 = case shown="False" w243 {
                            tunnel: w245 -> [w248 w249]
                            tunnel: [w247 w249] -> w244
                            frame False {
                              w246 = TRUE
                              n282 = Increment(x=w248) -> (x+1=w247:u16)
                              "Current trial #" <- w247
                              n283 = local write "VS busy"(w246) -> ()
                              n284 = local write "State busy"(w246) -> ()
                            }
                            frame True {
                            }
                          }
                        }
                      }
                      n285 = local read "Remote IP_Broadcast"() -> (w78:string)
                      n286 = local read "Remote port"() -> (w80:u16)
                      n287 = String To IP(1:w78) -> (0:w79:u32)
                      n288 = UDP Write(address=w79, port or service name=w80, connection ID=w76, data in=w67, 8:w77) -> (error out=w75:errorcluster, 3:w74:refnum<k16>)  [unwired: 1 in]
                    }
                    frame True {
                      n289 = stacked-sequence {
                        seq-local: [w270 _] -> [_ w366]
                        seq-local: [w269 _] -> [_ w367]
                        tunnel: w260 -> [w286 _]
                        tunnel: w259 -> [w277 _]
                        tunnel: w258 -> [w276 _]
                        tunnel: [_ w361] -> w257
                        tunnel: w256 -> [w275 _]
                        tunnel: [_ w358] -> w255
                        tunnel: [w263 _] -> w254
                        tunnel: [w271 _] -> w253
                        tunnel: w252 -> [_ w355]
                        tunnel: [_ w353] -> w251
                        frame #0 {
                          n290 = local read "Manually give shock"() -> (w296:bool)
                          n291 = local read "Manually give water"() -> (w298:bool)
                          n292 = local read "Shock refractory period (ms)"() -> (w306:u32)
                          n293 = local read "Lick threshold (V)"() -> (w287:fxp<+,32,16>)
                          n294 = local read "Water refractory period (ms)"() -> (w308:u32)
                          n295 = local read "VS threshold (V)"() -> (w267:fxp<+,32,16>)
                          n296 = local read "Allow timeout"() -> (w300:bool)
                          n297 = local read "Reward start delay (ms)"() -> (w310:u32)
                          n298 = local read "Allow shock"() -> (w302:bool)
                          n299 = local read "Save data"() -> (w294:bool)
                          n300 = local read "Shock duration (ms)"() -> (w307:u32)
                          n301 = local read "Track eye"() -> (w303:bool)
                          n302 = local read "Water duration (ms)"() -> (w309:u32)
                          n303 = local read "Reward period (ms)"() -> (w311:u32)
                          n304 = local read "Trial timeout (ms)"() -> (w305:u32)
                          n305 = Boolean To (0,1)(Boolean=w303) -> (0, 1=w304:i16)
                          n306 = Boolean To (0,1)(Boolean=w302) -> (0, 1=w301:i16)
                          n307 = Boolean To (0,1)(Boolean=w300) -> (0, 1=w299:i16)
                          n308 = Boolean To (0,1)(Boolean=w298) -> (0, 1=w297:i16)
                          n309 = Boolean To (0,1)(Boolean=w296) -> (0, 1=w295:i16)
                          n310 = Boolean To (0,1)(Boolean=w294) -> (0, 1=w293:i16)
                          n311 = To Single Precision Float(number=w287) -> (single precision float=w288:sgl)
                          n312 = To Single Precision Float(number=w267) -> (single precision float=w266:sgl)
                          n313 = local read "Give reward"() -> (w265:bool)
                          n314 = Boolean To (0,1)(Boolean=w265) -> (0, 1=w264:i16)
                          n315 = Build Array "Beh parameters"(w311, w310, w309, w308, w307, w306, w305, w288, w304, w301, w299, w297, w295, w293, w266, w264) -> (w271:sgl[])
                          n316 = Subtract(x=w271, y=w286) -> (x-y=w292:dbl[])
                          n317 = Absolute Value(x=w292) -> (abs(x)=w290:dbl[])
                          n318 = Less?(x=w290, y=1e-06) -> (x < y?=w289:bool[])
                          n319 = for {
                            tunnel: w289 -> [w326] mode=indexing
                            tunnel: w271 -> [w325] mode=indexing
                            shift-right: [w323] -> w272
                            shift-left: "" -> [w324]
                            i -> [w327]
                            n320 = case shown="False" w326 {
                              tunnel: w327 -> [w335 _]
                              tunnel: w325 -> [w333 _]
                              tunnel: w324 -> [w330 w352]
                              tunnel: [w328 w352] -> w323
                              frame False {
                                n321 = case shown="0, Default" w335 {
                                tunnel: ["rwp" "rwd" "wdr" "wre" "shd" "shr" "tto" "lkt" "etk" "ash" "ato" "gwt" "gsh" "sav" "vst" "rew"] -> w329
                                frame 0, Default {
                                }
                                frame 1 {
                                }
                                frame 2 {
                                }
                                frame 3 {
                                }
                                frame 4 {
                                }
                                frame 5 {
                                }
                                frame 6 {
                                }
                                frame 7 {
                                }
                                frame 8 {
                                }
                                frame 9 {
                                }
                                frame 10 {
                                }
                                frame 11 {
                                }
                                frame 12 {
                                }
                                frame 13 {
                                }
                                frame 14 {
                                }
                                frame 15 {
                                }
                                }
                                n322 = Format Value(format string="%.3f", value (0)=w333) -> (output string=w331:string)  [unwired: 1 in]
                                n323 = call <vilib>:"Space Constant.vi"() -> ("String"=w332:string)
                                n324 = Concatenate Strings(w330, w329, w332, w331, w332) -> (w328:string)
                              }
                              frame True {
                              }
                            }
                          }
                          n325 = String Length(string=w272) -> (length=w273:i32)
                          n326 = Not Equal To 0?(x=w273) -> (x != 0?=w274:bool)
                          n327 = case shown="True" w274 {
                            tunnel: w276 -> [w312 w318]
                            tunnel: [w312 w317] -> w269
                            tunnel: w275 -> [w313 w316]
                            tunnel: [w313 w315] -> w270
                            tunnel: w272 -> [_ w314]
                            frame False {
                            }
                            frame True {
                              n328 = local read "Remote IP_Broadcast"() -> (w319:string)
                              n329 = local read "Remote port"() -> (w321:u16)
                              n330 = String To IP(1:w319) -> (0:w320:u32)
                              n331 = UDP Write(address=w320, port or service name=w321, connection ID=w316, data in=w314, 8:w318) -> (error out=w317:errorcluster, 3:w315:refnum<k16>)  [unwired: 1 in]
                            }
                          }
                          n332 = local read "Total number of trials"() -> (w268:i32)
                          n333 = local read "Current trial #"() -> (w281:u16)
                          n334 = local read "run-stop"() -> (w280:bool)
                          n335 = local read "State Missed"() -> (w283:bool)
                          n336 = local read "VS missed"() -> (w282:bool)
                          n337 = Not(x=w280) -> (.not. x?=w279:bool)
                          n338 = Equal?(x=w281, y=w268) -> (x = y?=w284:bool)
                          n339 = Compound Arithmetic op=OR(w282, w283, w284) -> (w278:bool)
                          n340 = Compound Arithmetic op=OR(w278, w279, w277) -> (w263:bool)
                          n341 = case shown="True" w263 {
                            frame False {
                            }
                            frame True {
                              w322 = FALSE
                              n342 = local write "Running!"(w322) -> ()
                              n343 = local write "run-stop"(w322) -> ()
                            }
                          }
                        }
                        frame #1 {
                          n344 = UDP Read(connection ID=w366, timeout ms (25000)=0, 8:w367) -> (data out=w354:string, error out=w362:errorcluster, 3:w358:refnum<k16>, 6:w356:u32)  [unwired: 1 in, 1 out]
                          n345 = Unbundle By Name(w362) -> ("code"=w363:i32)
                          n346 = Equal?(x=w363, y=56) -> (x = y?=w365:bool)
                          n347 = case shown="True" w365 {
                            tunnel: w362 -> [w407 _]
                            tunnel: [w407 errorcluster {"status"=FALSE, "code"=0, "source"=""} ("error out")] -> w361
                            frame False {
                            }
                            frame True {
                            }
                          }
                          n348 = String Length(string=w354) -> (length=w360:i32)
                          n349 = Not Equal To 0?(x=w360) -> (x != 0?=w359:bool)
                          n350 = case shown="True" w359 {
                            tunnel: w356 -> [_ w372]
                            tunnel: w355 -> [w368 w371]
                            tunnel: w354 -> [_ w376]
                            tunnel: [w368 w369] -> w353
                            frame False {
                            }
                            frame True {
                              (unwired) -1.0 ("default value 2")
                              (unwired) "no" ("default value 1")
                              n351 = Scan From String(format string="%s %f ", input string=w376, initial scan location=u32 0) -> (output 1=w373:string, output 2=w370:dbl)  [unwired: 3 in, 3 out]
                              n352 = case shown="\"TrlDone\", Default" w373 {
                                tunnel: w372 -> [w384]
                                tunnel: w371 -> [w377]
                                tunnel: w370 -> [w379]
                                tunnel: [w377] -> w369
                                frame "TrlDone", Default {
                                n353 = local read "Remote IP_State machine"() -> (w381:string)
                                n354 = IP To String(1:TRUE ("dot notation? (F)"), 2:w384) -> (0:w378:string)
                                "Originating IP" <- w378
                                n355 = Match True/False String(2:"" ("false string"), 3:w381, 4:w378) -> (0:w380:bool)  [unwired: 1 out]
                                n356 = case shown="False" w380 {
                                tunnel: w377 -> [w385 w404]
                                tunnel: w379 -> [w386 w405]
                                tunnel: w378 -> [w390 _]
                                frame False {
                                n357 = local read "Remote IP_Visual stimulation"() -> (w388:string)
                                n358 = Match True/False String(2:"" ("false string"), 3:w388, 4:w390) -> (0:w387:bool)  [unwired: 1 out]
                                n359 = case shown="True" w387 {
                                tunnel: w386 -> [_ w395]
                                tunnel: w385 -> [_ w394]
                                frame False {
                                "Error 2" <- "Unknown source Error"
                                }
                                frame True {
                                n360 = Subtract(x=w395, y=w394) -> (x-y=w398:dbl)
                                n361 = global write "Global 1.vi" "camera stop"(TRUE ("dot notation? (F)")) -> ()
                                n362 = Absolute Value(x=w398) -> (abs(x)=w397:dbl)
                                n363 = local write "VS busy"(FALSE) -> ()
                                n364 = Greater?(x=w397, y=1e-06) -> (0:→"VS missed":bool)
                                }
                                }
                                }
                                frame True {
                                n365 = Subtract(x=w405, y=w404) -> (x-y=w403:dbl)
                                n366 = local write "State busy"(FALSE) -> ()
                                n367 = Absolute Value(x=w403) -> (abs(x)=w402:dbl)
                                n368 = Greater?(x=w402, y=1e-06) -> (0:→"State Missed":bool)
                                }
                                }
                                }
                              }
                              "Incoming data" <- w376
                            }
                          }
                        }
                      }
                    }
                  }
                  n369 = node-c288() -> ()  [unwired: 1 in, 1 out]
                }
                n370 = node-c288(w38) -> ()  [unwired: 1 out]
                n371 = To Single Precision Float(number=w28) -> (single precision float=w23:sgl[][])
                n372 = local read "Save data"() -> (w26:bool)
                n373 = UDP Close(connection ID=w17, 8:w16) -> (error out=w21:errorcluster)  [unwired: 1 out]
                n374 = case shown="True" w26 {
                  tunnel: w25 -> [w413 w429]
                  tunnel: w24 -> [_ w428]
                  tunnel: w23 -> [_ w420]
                  tunnel: [w413 w417] -> w20
                  tunnel: w15 -> [_ w416]
                  frame False {
                  }
                  frame True {
                    n375 = Add(x=w416, y=2) -> (x+y=w414:i32)
                    n376 = Multiply(x=w414, y=4) -> (x*y=w425:i32)
                    n377 = Set File Position(offset (in bytes) (0)=w425, refnum=w428, from (0:start)=enum16{"start", "end", "current"}."start", error in=w429) -> (refnum out=w422:refnum<file>, error out=w423:errorcluster)
                    n378 = Write to Binary File(file (use dialog)=w422, data=w420, error in=w423, 5:FALSE ("prepend array or string size? (T)"), 9:T5."little-endian" ("byte order (0:big-endian, network order)")) -> (refnum out=w418:refnum<file>, error out=w419:errorcluster)  [unwired: 1 in, 1 out]
                    n379 = Close File(refnum=w418, error in=w419) -> (error out=w417:errorcluster)  [unwired: 1 out]
                  }
                }
                n380 = Merge Errors(w21, w20) -> (w19:errorcluster)
                n381 = stacked-sequence {
                  tunnel: w19 -> [w40]
                  frame #0 {
                    n382 = call <vilib>:"Simple Error Handler.vi"("error in (no error)"=w40) -> ()  [unwired: 4 in, 5 out]
                  }
                }
              }
              frame 2 {
              }
            }
          }
          frame #2 {
            n383 = Wait (ms)(milliseconds to wait=u32 100) -> ()  [unwired: 1 out]
          }
        }
      }
    }
  }
